vi "EditorPDF openPDF.vi"(8 "error in (no error)":errorcluster, 11 "CreatePDF in":refnum<class "CreatePDF.lvclass">) -> (0 "error out":errorcluster, 3 "CreatePDF out":refnum<class "CreatePDF.lvclass">)   [LabVIEW 2018, in "CreatePDF.lvclass"]
uses:
  CreatePDF.lvclass
  <vilib>/Simplicity AI/SAI_PDF_API/Classes/Context/Controls/SAI_PDF_Type.ctl
  <vilib>/Simplicity AI/SAI_PDF_API/Classes/Context/Controls/SAI_PDF_File dialog mode.ctl
  CreatePDF.lvclass/CreatePDF.ctl
  <vilib>/Simplicity AI/SAI_PDF_API/Classes/Context/Context.lvclass
panel:
  in  "PDF Type":T1 items=["Normal", "PDF_A_1b"]
  in  "License Path":path
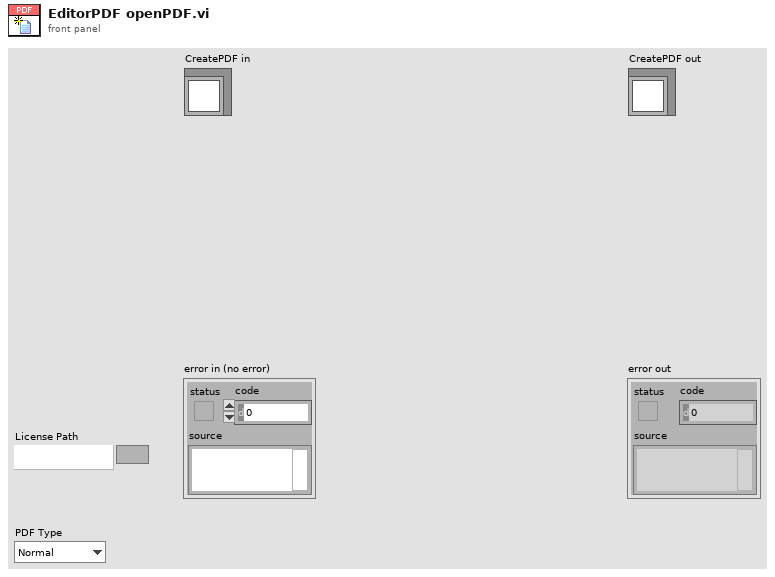
[diagram p1: front panel]
types:
  T1 = typedef "SAI_PDF_Toolkit.lvlib/Context.lvclass/SAI_PDF_Type.ctl" = i32
  T2 = typedef "SAI_PDF_Toolkit.lvlib/Context.lvclass/SAI_PDF_File dialog mode.ctl" = enum16{"Existing File", "New File"}
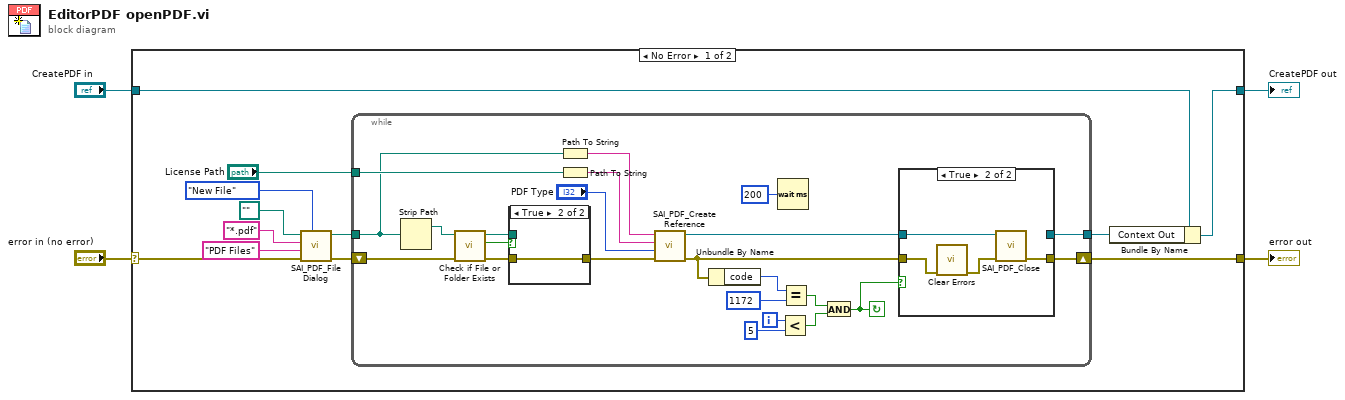
[diagram p0: block diagram]
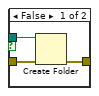
[diagram p3: hidden frame]
diagram:
  n1 = case shown="No Error" "error in (no error)" {
    selector: "error in (no error)" -> [w6 w51]
    tunnel: [w5 w51] -> w3
    tunnel: [w14 w50] -> w1
    tunnel: "CreatePDF in" -> [w16 w50]
    frame No Error {
      n2 = call <vilib>:"SAI_PDF_File Dialog.vi"("Mode"=SAI_PDF_File_dialog_mode."New File", "error in"=w6, "Pattern label"="PDF Files", "Pattern"="*.pdf", "Path In"=path "") -> ("error out"=w8:errorcluster, "Path Out"=w7:path)  [unwired: 5 out]
      n3 = while {
        tunnel: [w20] -> w15
        shift-right: [w23] -> w5
        shift-left: w8 -> [w18]
        tunnel: "License Path" -> [w24]
        tunnel: w7 -> [w17]
        i -> [w29]
        stop <- w21 continue-if-true
        n4 = Strip Path(path=w17) -> (stripped path=w39:path)  [unwired: 1 out]
        n5 = call <vilib>:"Check if File or Folder Exists.vi"("error in (no error)"=w18, "path"=w39) -> ("error out"=w37:errorcluster, "file or folder exists?"=w36:bool, "dup path"=w38:path)  [unwired: 7 out]
        n6 = case shown="True" w36 {
          tunnel: w38 -> [w48 _]
          tunnel: w37 -> [w47 w49]
          tunnel: [w46 w49] -> w32
          frame False {
            n7 = Create Folder(path (use dialog)=w48, error in=w47) -> (error out=w46:errorcluster)  [unwired: 3 out]
          }
          frame True {
          }
        }
        n8 = Path To String(path=w17) -> (string=w34:string)
        n9 = Path To String(path=w24) -> (string=w33:string)
        n10 = call <vilib>:"SAI_PDF_Create Reference.vi"("error in (no error)"=w32, "PDF Type"="PDF Type", "License Path"=w33, "File Path"=w34) -> ("error out"=w22:errorcluster, "PDF Context"=w19:refnum<class "Context.lvclass">)  [unwired: 6 out]
        n11 = Unbundle By Name(w22) -> ("code"=w31:i32)
        n12 = Wait (ms)(milliseconds to wait=u32 200) -> ()  [unwired: 1 out]
        n13 = Less?(x=w29, y=5) -> (x < y?=w26:bool)
        n14 = Equal?(x=w31, y=1172) -> (x = y?=w27:bool)
        n15 = And(x=w27, y=w26) -> (x .and. y?=w21:bool)
        n16 = case shown="True" w21 {
          tunnel: [w40 w44] -> w23
          tunnel: w22 -> [w40 w43]
          tunnel: [w41 _] -> w20
          tunnel: w19 -> [w41 w45]
          frame False {
          }
          frame True {
            n17 = call <vilib>:"Clear Errors.vi"("error in (no error)"=w43) -> ("error out"=w42:errorcluster)  [unwired: 5 in, 1 out]
            n18 = call <vilib>:"SAI_PDF_Close.vi"("error in"=w42, "Context In"=w45) -> ("error out"=w44:errorcluster)  [unwired: 9 out]
          }
        }
      }
      n19 = Bundle By Name(cluster=w16, "Context Out"=w15) -> (w14:refnum<class "CreatePDF.lvclass">)
    }
    frame Error {
    }
  }
  "error out" <- w3
  "CreatePDF out" <- w1
